vi "DER Randomize Infos.vi"(10 "DeviceID":T2) -> (3 "DER Info Array":T1[](array[typedef]))   [LabVIEW 2018, in "IED Test Framework.lvlib" / "IED Test.lvclass"]
uses:
  IED Test.lvclass
  <vilib>/ORNL/CSEISMIC DDS/CSEISMIC DDS Base/Data Types/Controls/DeviceID.ctl
  <vilib>/ORNL/CSEISMIC DDS/CSEISMIC DDS Base/Data Types/DER_Info.ctl
  <vilib>/ORNL/CSEISMIC DDS/CSEISMIC DDS Base/CSEISMIC DDS.lvclass
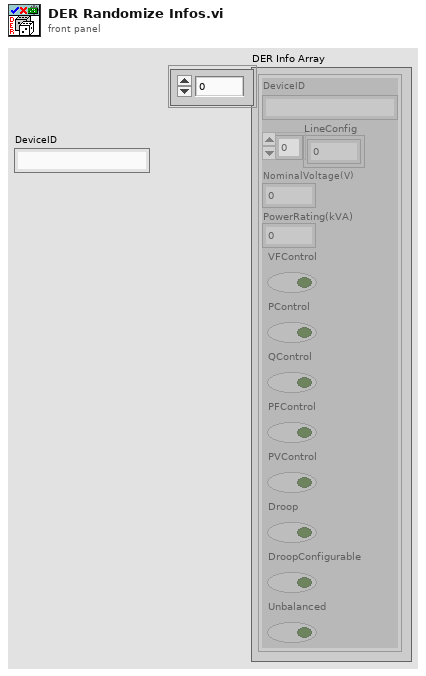
[diagram p1: front panel]
types:
  T1 = typedef "CSEISMIC DDS.lvlib/CSEISMIC DDS.lvclass/DER_Info.ctl" = cluster{"DeviceID":T2, "LineConfig":u8[], "NominalVoltage(V)":dbl, "PowerRating(kVA)":dbl, "VFControl":bool, "PControl":bool, "QControl":bool, "PFControl":bool, "PVControl":bool, "Droop":bool, "DroopConfigurable":bool, "Unbalanced":bool}
  T2 = typedef "CSEISMIC DDS.lvlib/CSEISMIC DDS.lvclass/DeviceID.ctl" = string
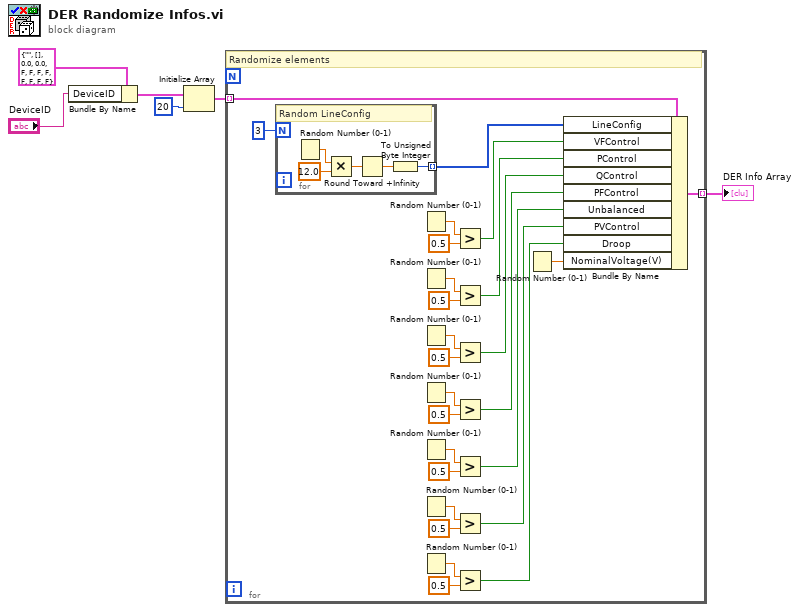
[diagram p0: block diagram]
diagram:
  n1 = Bundle By Name(cluster=T1 {"DeviceID"="", "LineConfig"=[], "NominalVoltage(V)"=0.0, "PowerRating(kVA)"=0.0, "VFControl"=FALSE, "PControl"=FALSE, "QControl"=FALSE, "PFControl"=FALSE, "PVControl"=FALSE, "Droop"=FALSE, "DroopConfigurable"=FALSE, "Unbalanced"=FALSE} ("DER_Info"), "DeviceID"="DeviceID") -> (w6:T1)
  n2 = Initialize Array(w6, 20 ("dimension size")) -> (w3:T1[])
  n3 = for {
    tunnel: w3 -> [w32] mode=indexing
    tunnel: [w31] -> w1 mode=indexing
    # "Randomize elements"
    n4 = for {
      N: 3 -> [_]
      tunnel: [w33] -> w14 mode=indexing
      # "Random LineConfig"
      n5 = Random Number (0-1)() -> (number: 0 to 1=w37:dbl)
      n6 = Multiply(x=w37, y=12.0) -> (x*y=w35:dbl)
      n7 = Round Toward +Infinity(x=w35) -> (ceil(x): smallest int >= x=w34:dbl)
      n8 = To Unsigned Byte Integer(number=w34) -> (unsigned 8bit integer=w33:u8)
    }
    n9 = Random Number (0-1)() -> (number: 0 to 1=w30:dbl)
    n10 = Random Number (0-1)() -> (number: 0 to 1=w25:dbl)
    n11 = Random Number (0-1)() -> (number: 0 to 1=w24:dbl)
    n12 = Random Number (0-1)() -> (number: 0 to 1=w21:dbl)
    n13 = Random Number (0-1)() -> (number: 0 to 1=w18:dbl)
    n14 = Random Number (0-1)() -> (number: 0 to 1=w13:dbl)
    n15 = Random Number (0-1)() -> (number: 0 to 1=w9:dbl)
    n16 = Greater?(x=w30, y=0.5) -> (0:w29:bool)
    n17 = Greater?(x=w25, y=0.5) -> (0:w23:bool)
    n18 = Greater?(x=w24, y=0.5) -> (0:w22:bool)
    n19 = Greater?(x=w21, y=0.5) -> (0:w17:bool)
    n20 = Greater?(x=w18, y=0.5) -> (0:w16:bool)
    n21 = Greater?(x=w13, y=0.5) -> (0:w11:bool)
    n22 = Greater?(x=w9, y=0.5) -> (0:w8:bool)
    n23 = Random Number (0-1)() -> (number: 0 to 1=w7:dbl)
    n24 = Bundle By Name(cluster=w32, "LineConfig"=w14, "VFControl"=w29, "PControl"=w23, "QControl"=w22, "PFControl"=w17, "Unbalanced"=w16, "PVControl"=w11, "Droop"=w8, "NominalVoltage(V)"=w7) -> (w31:T1)
  }
  "DER Info Array" <- w1
